vi "Event Handler.vi"(8 "error in (no error)":errorcluster, 10 "Stop Event Handler":refnum<user-event>, 11 "AdjustableMulticolumnListbox in":refnum<class "AdjMCLB.lvclass">) -> (0 "error out":errorcluster)   [LabVIEW 2020, in "AdjMCLB.lvclass"]
doc: "The <b>Event Handler VI</b> is a dynamic dispatch VI that should be overwritten if events are needed to create the enhanced QControl. \n\nBy inheriting from the main Control.lvclass the overwritten <b>Event Handler VI</b> will be launched asynchronously in the initialization of the QControl.\n<b> </b> <b> </b>\n©2016 Q Software Innovations, LLC (QSI)\nwritten by Quentin Alldredge\nproduced in LabVIEW 2015\n\nsupport@qsoftwareinnovations.com\nwww.qsoftwareinnovations.com\n\nAll rights reserved.\n\nRedistribution and use in source and binary forms, with or without modification, are permitted provided that the following conditions are met:\n\n * Redistributions of source code must retain the above copyright notice, this list of conditions and the following disclaimer.\n * Redistributions in binary form must reproduce the above copyright notice, this list of conditions and the following disclaimer in the documentation and/or other materials provided with the distribution.\n * Neither the name of Q Software Innovations, LLC. nor the names of its contributors may be used to endorse or promote products derived from this software without specific prior written permission.\n\nTHIS SOFTWARE IS PROVIDED BY THE COPYRIGHT HOLDERS AND CONTRIBUTORS \"AS IS\" AND ANY EXPRESS OR IMPLIED WARRANTIES, INCLUDING, BUT NOT LIMITED TO, THE IMPLIED WARRANTIES OF MERCHANTABILITY AND FITNESS FOR A PARTICULAR PURPOSE ARE DISCLAIMED. IN NO EVENT SHALL THE COPYRIGHT OWNER OR CONTRIBUTORS BE LIABLE FOR ANY DIRECT, INDIRECT, INCIDENTAL, SPECIAL, EXEMPLARY, OR CONSEQUENTIAL DAMAGES (INCLUDING, BUT NOT LIMITED TO, PROCUREMENT OF SUBSTITUTE GOODS OR SERVICES; LOSS OF USE, DATA, OR PROFITS; OR BUSINESS INTERRUPTION) HOWEVER CAUSED AND ON ANY THEORY OF LIABILITY, WHETHER IN CONTRACT, STRICT LIABILITY, OR TORT (INCLUDING NEGLIGENCE OR OTHERWISE) ARISING IN ANY WAY OUT OF THE USE OF THIS SOFTWARE, EVEN IF ADVISED OF THE POSSIBILITY OF SUCH DAMAGE."
uses:
  AdjMCLB.lvclass
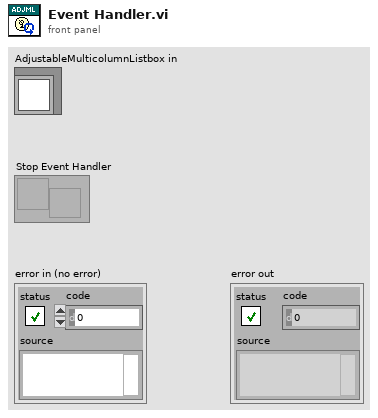
[diagram p1: front panel]
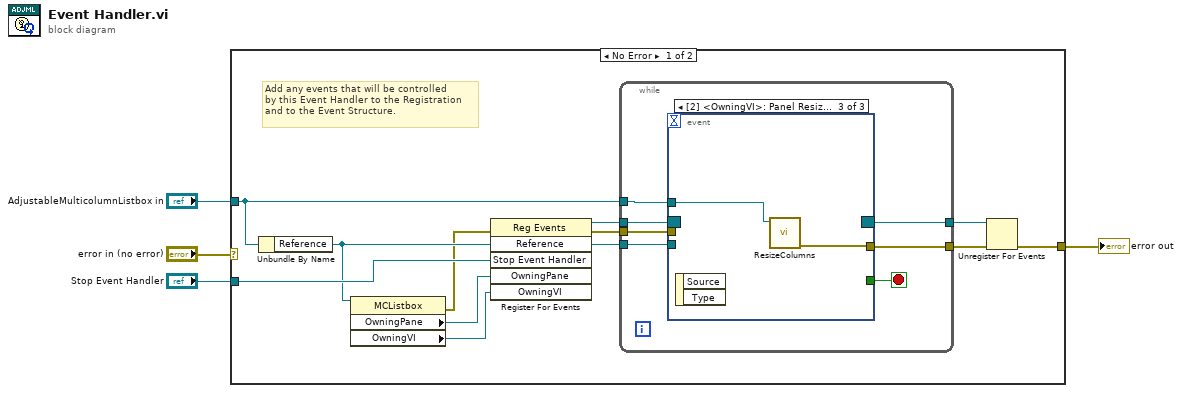
[diagram p0: block diagram]
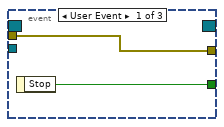
[diagram p2: hidden frame]
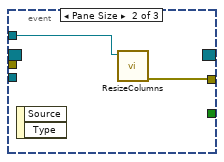
[diagram p3: hidden frame]
diagram:
  n1 = case shown="No Error" "error in (no error)" {
    selector: "error in (no error)" -> [_ w29]
    tunnel: [w12 w29] -> w3
    tunnel: "AdjustableMulticolumnListbox in" -> [w10 _]
    tunnel: "Stop Event Handler" -> [w9 _]
    frame No Error {
      # "Add any events that will be controlled\nby this Event Handler to the Registration\nand to the Event Structure."
      n2 = Unbundle By Name(w10) -> ("Reference"=w8:refnum<vi>)
      n3 = property class="MCListbox"(reference=w8) -> (error out=w5:errorcluster, "OwningPane"=w7:refnum<vi>, "OwningVI"=w6:refnum<vi>)  [unwired: 1 in, 1 out]
      n4 = register-events(error in=w5, w8, w9, w7, w6) -> (reference out=w15:refnum<event-registration>, error out=w14:errorcluster)  [unwired: 1 in]
      n5 = while {
        tunnel: w15 -> [w22]
        tunnel: w14 -> [w21]
        tunnel: [w17] -> w13
        tunnel: [w19] -> w11
        tunnel: w8 -> [w18]
        tunnel: w10 -> [w16]
        stop <- w20 stop-if-true
        n6 = event shown="[2] <OwningVI>: Panel Resize" {
          selector: w22 -> [_ _ _]
          dyn-events: [_ _ _] -> w19
          timeout: _ -> [_ _ _]
          tunnel: w21 -> [w24 _ _]
          tunnel: [w24 w25 w28] -> w17
          tunnel: [w23 _ _] -> w20
          tunnel: w18 -> [_ _ _]
          tunnel: w16 -> [_ w26 w27]
          event User Event {
            n7 = event-data() -> ("Stop"=w23:bool)  [unwired: 1 in]
          }
          event Pane Size {
            n8 = event-data() -> ()  [unwired: 1 in, 2 out]
            n9 = call "ResizeColumns.vi"("AdjustableMulticolumnListbox in"=w26) -> ("error out"=w25:errorcluster)  [unwired: 9 in, 1 out]
          }
          event Panel Resize {
            n10 = event-data() -> ()  [unwired: 1 in, 2 out]
            n11 = call "ResizeColumns.vi"("AdjustableMulticolumnListbox in"=w27) -> ("error out"=w28:errorcluster)  [unwired: 9 in, 1 out]
          }
        }
      }
      n12 = Unregister For Events(event registration refnum=w11, error in=w13) -> (error out=w12:errorcluster)
    }
    frame Error {
    }
  }
  "error out" <- w3
